vi "Scan_AlignImage.vi"(5 "slow axis":dbl, 6 "fast axis":dbl, 7 "Axis":enum32{"x-y", "x-z", "y-x", "y-z", "z-x", "z-y"}(ring), 8 "Scanner XYZ":T1) -> (0 "Image Y end":dbl, 1 "Image Y start":dbl, 2 "Image X end":dbl, 3 "Image X start":dbl)   [LabVIEW 2009]
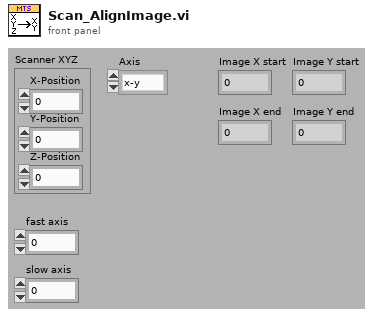
[diagram p1: front panel]
types:
  T1 = cluster{"X-Position":dbl, "Y-Position":dbl, "Z-Position":dbl}
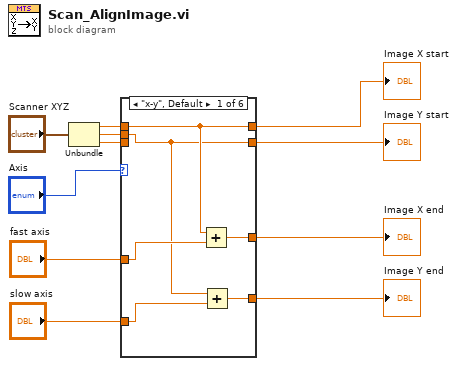
[diagram p0: block diagram]
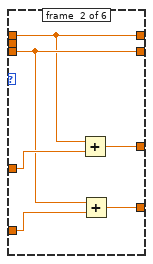
[diagram p2: hidden frame]
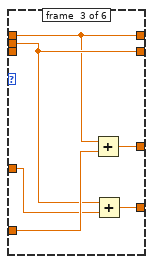
[diagram p3: hidden frame]
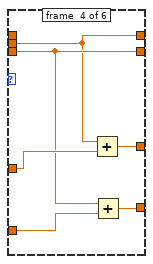
[diagram p4: hidden frame]
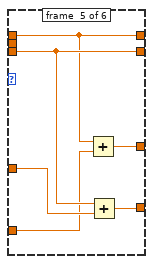
[diagram p5: hidden frame]
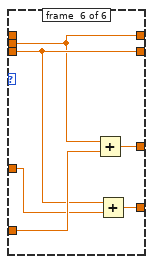
[diagram p6: hidden frame]
diagram:
  n1 = Unbundle("Scanner XYZ") -> ("X-Position"=w7:dbl, "Y-Position"=w8:dbl, "Z-Position"=w9:dbl)
  n2 = case shown="\"x-y\", Default" "Axis" {
    tunnel: w7 -> [w15 w18 w24 _ w37 _]
    tunnel: w8 -> [w12 _ w25 w30 _ w42]
    tunnel: w9 -> [_ w19 _ w31 w38 w43]
    tunnel: [w15 w18 w24 w30 w37 w42] -> w10
    tunnel: [w12 w19 w25 w31 w38 w43] -> w11
    tunnel: [w17 w23 w28 w35 w41 w46] -> w4
    tunnel: [w16 w22 w29 w34 w40 w47] -> w3
    tunnel: "slow axis" -> [w13 w21 w27 w33 w36 w45]
    tunnel: "fast axis" -> [w14 w20 w26 w32 w39 w44]
    frame #0 {
      n3 = Add(x=w15, y=w14) -> (x+y=w17:dbl)
      n4 = Add(x=w12, y=w13) -> (x+y=w16:dbl)
    }
    frame #1 {
      n5 = Add(x=w18, y=w20) -> (x+y=w23:dbl)
      n6 = Add(x=w19, y=w21) -> (x+y=w22:dbl)
    }
    frame #2 {
      n7 = Add(x=w24, y=w27) -> (x+y=w28:dbl)
      n8 = Add(x=w25, y=w26) -> (x+y=w29:dbl)
    }
    frame #3 {
      n9 = Add(x=w30, y=w32) -> (x+y=w35:dbl)
      n10 = Add(x=w31, y=w33) -> (x+y=w34:dbl)
    }
    frame #4 {
      n11 = Add(x=w37, y=w36) -> (x+y=w41:dbl)
      n12 = Add(x=w38, y=w39) -> (x+y=w40:dbl)
    }
    frame #5 {
      n13 = Add(x=w42, y=w45) -> (x+y=w46:dbl)
      n14 = Add(x=w43, y=w44) -> (x+y=w47:dbl)
    }
  }
  "Image Y start" <- w11
  "Image X start" <- w10
  "Image Y end" <- w3
  "Image X end" <- w4
